vi "Download History Data.vi"(8 "error in (no error)":errorcluster caption="entrée d'erreur (pas d'erreur)", 10 "Min_Date":string="1990", 11 "Share en entrée":refnum<class "Stock.lvclass"> caption="DNL_LabVIEW Object in") -> (0 "error out":errorcluster caption="sortie d'erreur", 2 "Download OK":bool, 3 "Share en sortie":refnum<class "Stock.lvclass"> caption="DNL_LabVIEW Object out", 4 "counter":i32)   [LabVIEW 2012, in "Stock.lvclass"]
uses:
  Stock.lvclass
  Stock_Data.ctl
  Stock.lvclass/Stock.ctl
  <vilib>/httpClient/LabVIEWHTTPClient.lvlib
panel:
  out "Tableau":T1[](array[typedef])
  out "header":string[][](array[string])
  out "End_Get":bool=TRUE
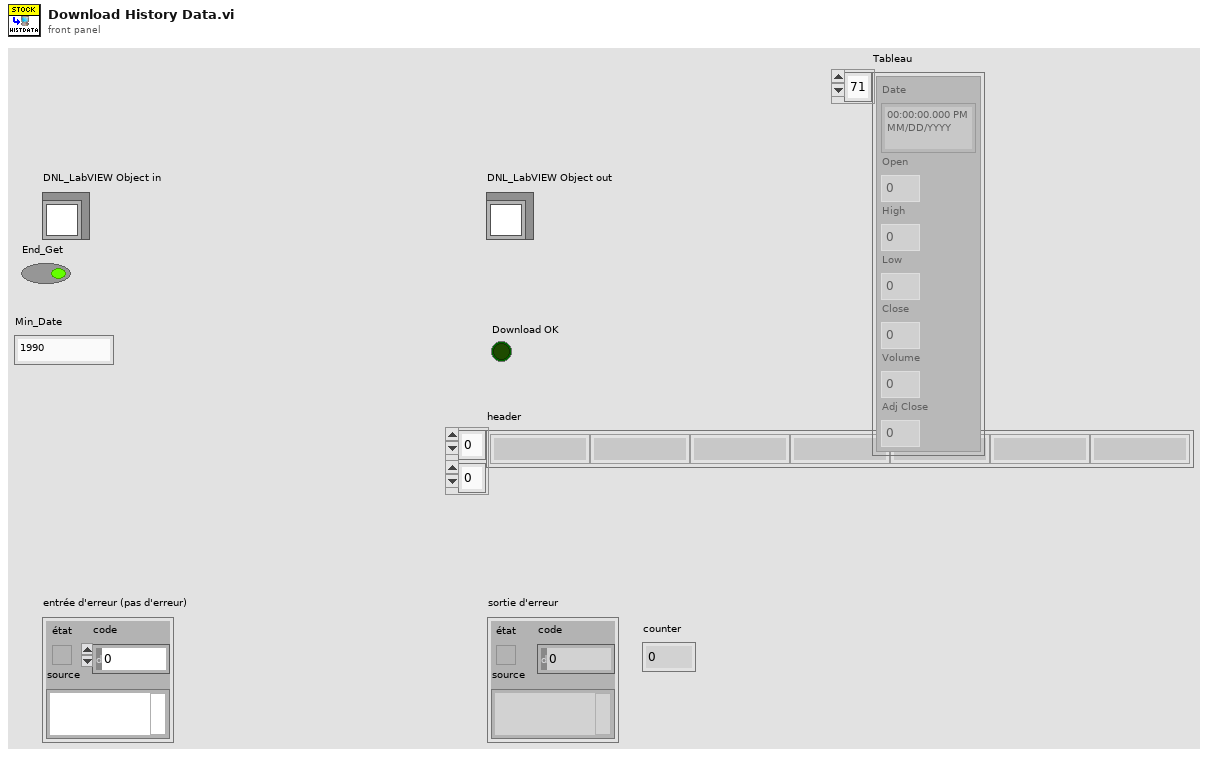
[diagram p1: front panel]
types:
  T1 = typedef "Stock_Data.ctl" = cluster{"Date":timestamp, "Open":dbl, "High":dbl, "Low":dbl, "Close":dbl, "Volume":dbl, "Adj Close":dbl}
  T2 = typedef "LabVIEWHTTPClient.lvlib/ClientHandle.ctl" = refnum<k1>
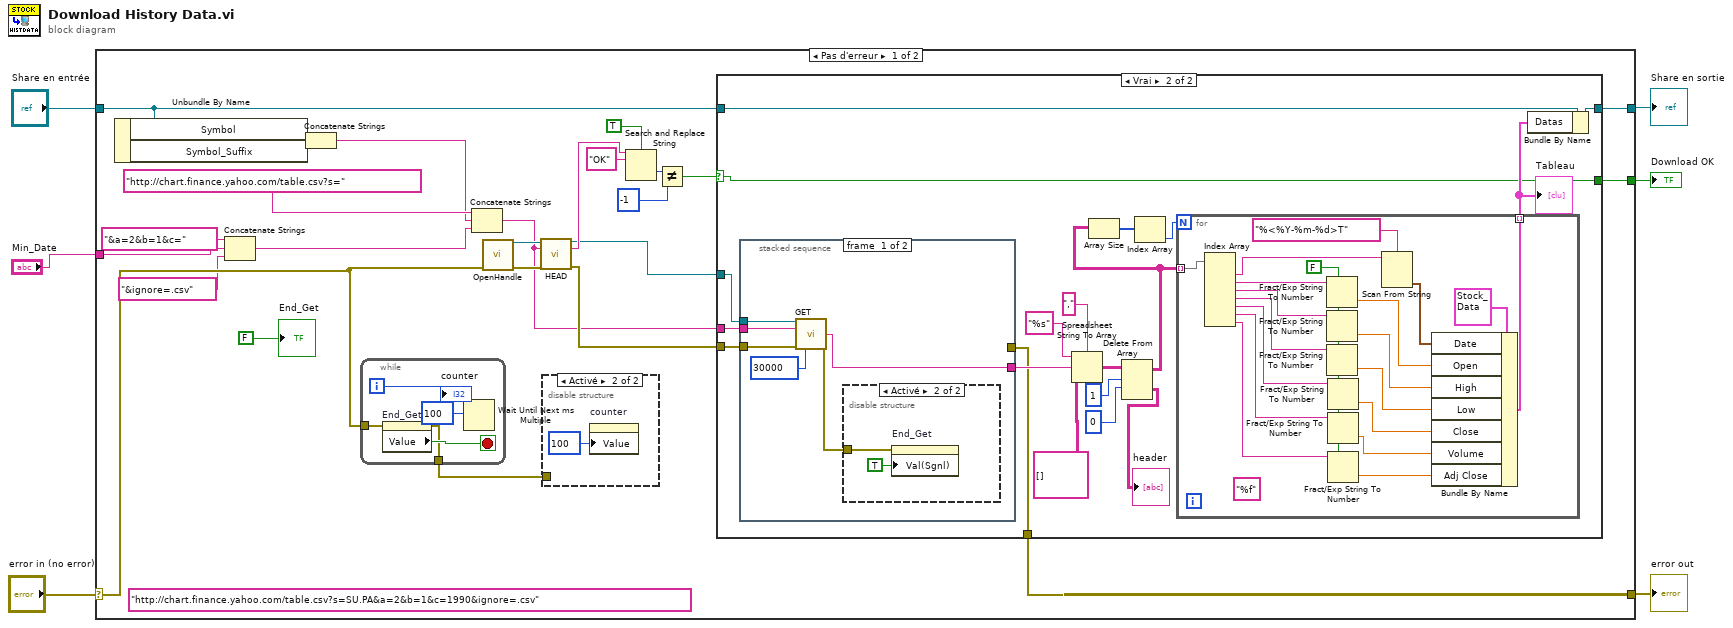
[diagram p0: block diagram]
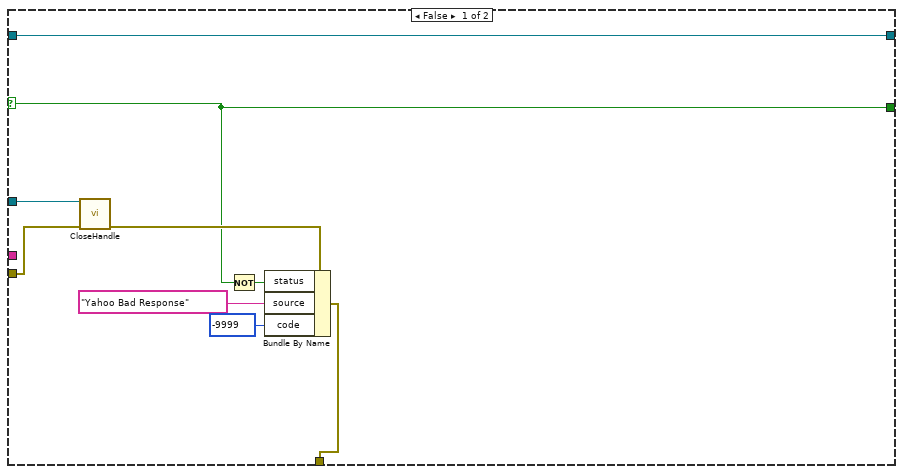
[diagram p3: hidden frame]
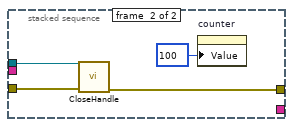
[diagram p5: hidden frame]
diagram:
  n1 = case shown="Pas d'erreur" "error in (no error)" {
    selector: "error in (no error)" -> [w16 w99]
    tunnel: [w19 w99] -> w5
    tunnel: [w13 w98] -> w3
    tunnel: "Share en entrée" -> [w14 w98]
    tunnel: [w12 _] -> w2
    tunnel: "Min_Date" -> [w9 _]
    frame No Error {
      (unwired) "http://chart.finance.yahoo.com/table.csv?s=SU.PA&a=2&b=1&c=1990&ignore=.csv"
      n2 = Unbundle By Name(w14) -> ("Symbol"=w32:string, "Symbol_Suffix"=w31:string)
      n3 = Concatenate Strings("&a=2&b=1&c=", w9, "&ignore=.csv") -> (w7:string)
      n4 = Concatenate Strings(w32, w31) -> (w11:string)
      n5 = while {
        tunnel: w16 -> [w35]
        tunnel: [w34] -> w15
        i -> [w38]
        stop <- w37 stop-if-true
        n6 = property on="End_Get" class="Bool (strict)"(error in=w35) -> (error out=w34:errorcluster, "Value"=w37:bool)  [unwired: 1 in, 1 out]
        n7 = Wait Until Next ms Multiple(millisecond multiple=u32 100 ("n millisecondes")) -> ()  [unwired: 1 out]
        "counter" <- w38
      }
      n8 = Concatenate Strings("http://chart.finance.yahoo.com/table.csv?s=", w11, w7) -> (w18:string)
      n9 = call <vilib>:"OpenHandle.vi"("error in (no error)"=w16) -> ("client handle out"=w25:T2, "error out"=w24:errorcluster)  [unwired: 13 in]
      n10 = call <vilib>:"HEAD.vi"("client handle"=w25, "url"=w18, "error in (no error)"=w24) -> ("client handle out"=w20:T2, "headers"=w23:string, "error out"=w21:errorcluster)  [unwired: 10 in]
      n11 = disable-structure shown="Activé" {
        disable-tunnel: w15 -> [_ _]
        frame Disabled {
        }
        frame Enabled {
          n12 = property on="counter" class="NumNb (strict)"("Value"=100 ("counter")) -> ()  [unwired: 2 in, 2 out]
        }
      }
      n13 = Search and Replace String(case sensitive?=TRUE ("ignorer la casse ? (F)"), input string=w23, search string="OK" ("chaîne recherchée")) -> (offset past replacement=w27:i32)  [unwired: 5 in, 3 out]
      n14 = Not Equal?(x=w27, y=-1) -> (x != y?=w22:bool)
      n15 = case shown="Vrai" w22 {
        selector: w22 -> [w39 w48]
        tunnel: [w47 w59] -> w19
        tunnel: w21 -> [w42 w63]
        tunnel: w20 -> [w43 w62]
        tunnel: w18 -> [_ w60]
        tunnel: w14 -> [w40 w51]
        tunnel: [w40 w55] -> w13
        tunnel: [w39 w48] -> w12
        frame False {
          n16 = call <vilib>:"CloseHandle.vi"("client handle"=w43, "error in (no error)"=w42) -> ("error out"=w41:errorcluster)  [unwired: 13 in]
          n17 = Not(x=w39) -> (.not. x?=w46:bool)
          n18 = Bundle By Name(cluster=w41, "status"=w46, "source"="Yahoo Bad Response" ("chaîne recherchée"), "code"=-9999) -> (w47:errorcluster)
        }
        frame True {
          n19 = stacked-sequence {
            tunnel: w63 -> [w90 w96]
            tunnel: w62 -> [w89 w97]
            tunnel: [w88 _] -> w61
            tunnel: w60 -> [w87 _]
            tunnel: [_ w95] -> w59
            frame #0 {
              n20 = call <vilib>:"GET.vi"("client handle"=w89, "url"=w87, "error in (no error)"=w90, "timeout (10000)"=30000) -> ("body"=w88:string, "error out"=w86:errorcluster)  [unwired: 8 in, 2 out]
              n21 = disable-structure shown="Activé" {
                disable-tunnel: w86 -> [_ w93]
                frame Disabled {
                }
                frame Enabled {
                  n22 = property on="End_Get" class="Bool (strict)"(error in=w93, "Val(Sgnl)"=TRUE ("Valeur (Signalisation)")) -> ()  [unwired: 1 in, 2 out]
                }
              }
            }
            frame #1 {
              n23 = call <vilib>:"CloseHandle.vi"("client handle"=w97, "error in (no error)"=w96) -> ("error out"=w95:errorcluster)  [unwired: 13 in]
              n24 = property on="counter" class="NumNb (strict)"("Value"=100 ("counter")) -> ()  [unwired: 2 in, 2 out]
            }
          }
          n25 = Spreadsheet String To Array(delimiter (Tab)=",", format string="%s", spreadsheet string=w61, array type (2D Dbl)=string[][] [] ("type de tableau (2D de dbl)")) -> (array=w58:string[][])
          n26 = Delete From Array(array=w58, length=1 ("longueur"), index (row)=0 ("indice (ligne)")) -> (deleted portion=→"header":string[][], array with subset deleted=w49:string[][])  [unwired: 1 in]
          n27 = Array Size(array=w49) -> (size(s)=w53:i32[])
          n28 = Index Array(array=w53) -> (element=w52:i32)  [unwired: 1 in]
          n29 = for {
            N: w52 -> [_]
            tunnel: w49 -> [w85] mode=indexing
            tunnel: [w84] -> w50 mode=indexing
            w69 = FALSE ("utiliser le séparateur décimal du système (V)")
            (unwired) "%f" ("chaîne de format")
            n30 = Index Array(array=w85) -> (element #1=w68:string, element #2=w75:string, element #3=w74:string, element #4=w73:string, element #5=w72:string, element #6=w71:string, element #7=w70:string)  [unwired: 7 in]
            n31 = Fract/Exp String To Number(use system decimal point (T)=w69, string=w75) -> (number=w83:dbl)  [unwired: 2 in, 1 out]
            n32 = Fract/Exp String To Number(use system decimal point (T)=w69, string=w74) -> (number=w82:dbl)  [unwired: 2 in, 1 out]
            n33 = Fract/Exp String To Number(use system decimal point (T)=w69, string=w73) -> (number=w81:dbl)  [unwired: 2 in, 1 out]
            n34 = Fract/Exp String To Number(use system decimal point (T)=w69, string=w72) -> (number=w80:dbl)  [unwired: 2 in, 1 out]
            n35 = Fract/Exp String To Number(use system decimal point (T)=w69, string=w71) -> (number=w79:dbl)  [unwired: 2 in, 1 out]
            n36 = Fract/Exp String To Number(use system decimal point (T)=w69, string=w70) -> (number=w78:dbl)  [unwired: 2 in, 1 out]
            n37 = Scan From String(format string="%<%Y-%m-%d>T" ("chaîne de format"), input string=w68) -> (output 1=w76:timestamp)  [unwired: 3 in, 3 out]
            n38 = Bundle By Name(cluster=T1 {"Date"=timestamp(0 s since 1904-01-01), "Open"=0.0, "High"=0.0, "Low"=0.0, "Close"=0.0, "Volume"=0.0, "Adj Close"=0.0} ("Share_Data"), "Date"=w76, "Open"=w83, "High"=w82, "Low"=w81, "Close"=w80, "Volume"=w79, "Adj Close"=w78) -> (w84:T1)
          }
          "Tableau" <- w50
          n39 = Bundle By Name(cluster=w51, "Datas"=w50) -> (w55:refnum<class "Stock.lvclass">)
        }
      }
      "End_Get" <- FALSE ("Valeur (Signalisation)")
    }
    frame Error {
    }
  }
  "error out" <- w5
  "Share en sortie" <- w3
  "Download OK" <- w2
